vi "Initialize.vi"(6 "optional":variant, 8 "error in":errorcluster, 11 "Channel in":refnum<class "Channel.lvclass">) -> (0 "error out":errorcluster, 3 "Node*":refnum<data-value>)   [LabVIEW 2013, in "Channel.lvclass"]
doc: "Initializes a node. Makes a data value reference of the node, sets the selfNode, and output the data value reference."
uses:
  Channel.lvclass
  xCE/xceNode/xceNode.lvclass
  xCE/xceDataNode/xceDataNode.lvclass
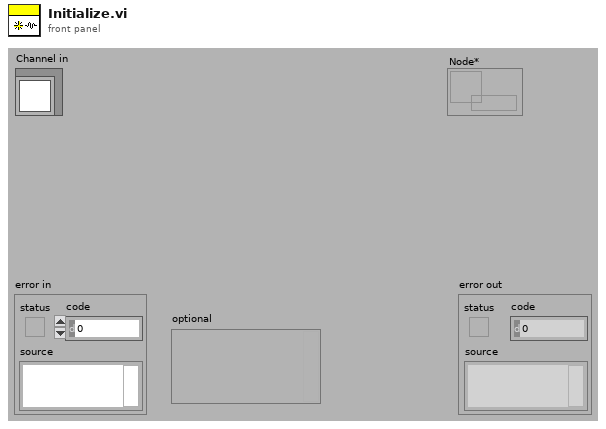
[diagram p1: front panel]
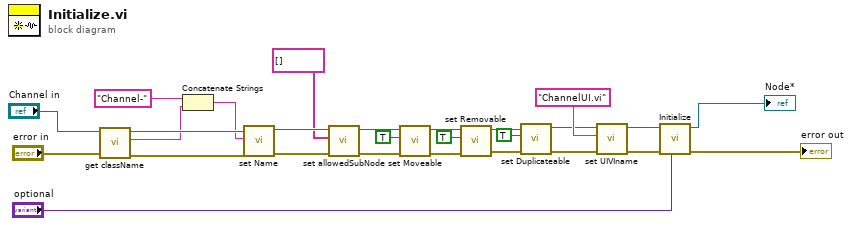
[diagram p0: block diagram]
diagram:
  n1 = call "get className.vi"("error in (no error)"="error in", "xceNode in"="Channel in") -> ("error out"=w6:errorcluster, "Class name"=w4:string, "xceNode out"=w7:refnum<class "Channel.lvclass">)  [unwired: 7 in]
  n2 = Concatenate Strings("Channel-" ("string"), w4) -> (w3:string)
  n3 = call "set Name.vi"("error in (no error)"=w6, "Name"=w3, "xceDataNode in"=w7) -> ("error out"=w12:errorcluster, "xceDataNode out"=w11:refnum<class "Channel.lvclass">)  [unwired: 7 in]
  n4 = call "set allowedSubNode.vi"("error in (no error)"=w12, "Allowed subNode[]"=string[] [], "xceDataNode in"=w11) -> ("error out"=w14:errorcluster, "xceDataNode out"=w13:refnum<class "Channel.lvclass">)  [unwired: 7 in]
  n5 = call "set Moveable.vi"("error in (no error)"=w14, "Moveable"=TRUE, "xceDataNode in"=w13) -> ("error out"=w17:errorcluster, "xceDataNode out"=w16:refnum<class "Channel.lvclass">)  [unwired: 7 in]
  n6 = call "set Removable.vi"("error in (no error)"=w17, "Removable"=TRUE, "xceDataNode in"=w16) -> ("error out"=w20:errorcluster, "xceDataNode out"=w19:refnum<class "Channel.lvclass">)  [unwired: 7 in]
  n7 = call "set Duplicateable.vi"("error in (no error)"=w20, "Duplicateable"=TRUE, "xceDataNode in"=w19) -> ("error out"=w23:errorcluster, "xceDataNode out"=w22:refnum<class "Channel.lvclass">)  [unwired: 7 in]
  n8 = call "set UIVIname.vi"("error in (no error)"=w23, "UI VI name"="ChannelUI.vi", "xceDataNode in"=w22) -> ("error out"=w1:errorcluster, "xceDataNode out"=w2:refnum<class "Channel.lvclass">)  [unwired: 7 in]
  n9 = call-parent "Initialize.vi"("optional"="optional", "error in"=w1, "xceDataNode in"=w2) -> ("error out"=→"error out":errorcluster, "Node*"=→"Node*":refnum<data-value>)  [unwired: 7 in]
